vi "LvIRKit_Main.vi"() -> ()   [LabVIEW 2014]
uses:
  <vilib>/Utility/sysdir.llb/System Directory Type.ctl
  <vilib>/Utility/miscctls.llb/LVPointTypeDef.ctl
  <vilib>/Platform/browser.llb/Open URL in Default Browser (string).vi
panel:
  in  "LvIRKit URL":bool
  in  "IRKit URL":bool
  out "title":string="LvIRKit"
  in  "Btn Edit":bool
  in  "Btn Dn":bool
  in  "Btn Up":bool
  in  "Btn Del":bool
  in  "Btn Add":bool
  in  "Btn Enter":bool
  in  "ButtonList":i32(listbox) caption="登録されているリモコンボタン"
  in  "Btn Dev Edit":bool
  in  "Btn Dev Dn":bool
  in  "Btn Dev Up":bool
  in  "Btn Dev Del":bool
  in  "Btn Dev Add":bool
  in  "DeviceList":i32(listbox) caption="IRKit"
  # "IRKit 非公式"
  # "LvIRKitについてはこちら"
  # "IRKitについてはこちら"
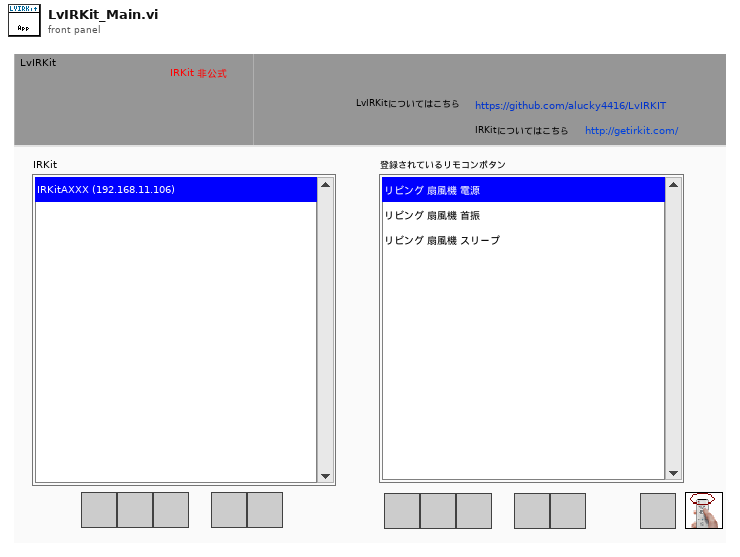
[diagram p1: front panel]
types:
  T1 = enum16{"Init", "Load", "Save", "Get", "Add", "Remove", "Replace", "Up", "Down"}
  T2 = typedef "System Directory Type.ctl" = i32
  T3 = typedef "LvIRKit_rsc_IRData_typedef.ctl" = cluster{"id":i32, "name":string, "irstr":string}
  T4 = typedef "LVPointTypeDef.ctl" = cluster{"Horizontal":i16, "Vertical":i16}
  T5 = cluster{bool, "include Ctrl key?":bool, string}[]
  T6 = enum32{"invalid app kind", "Development System", "Run Time System", "Student Edition", "Embedded LabVIEW", "Evaluation", "Custom"}
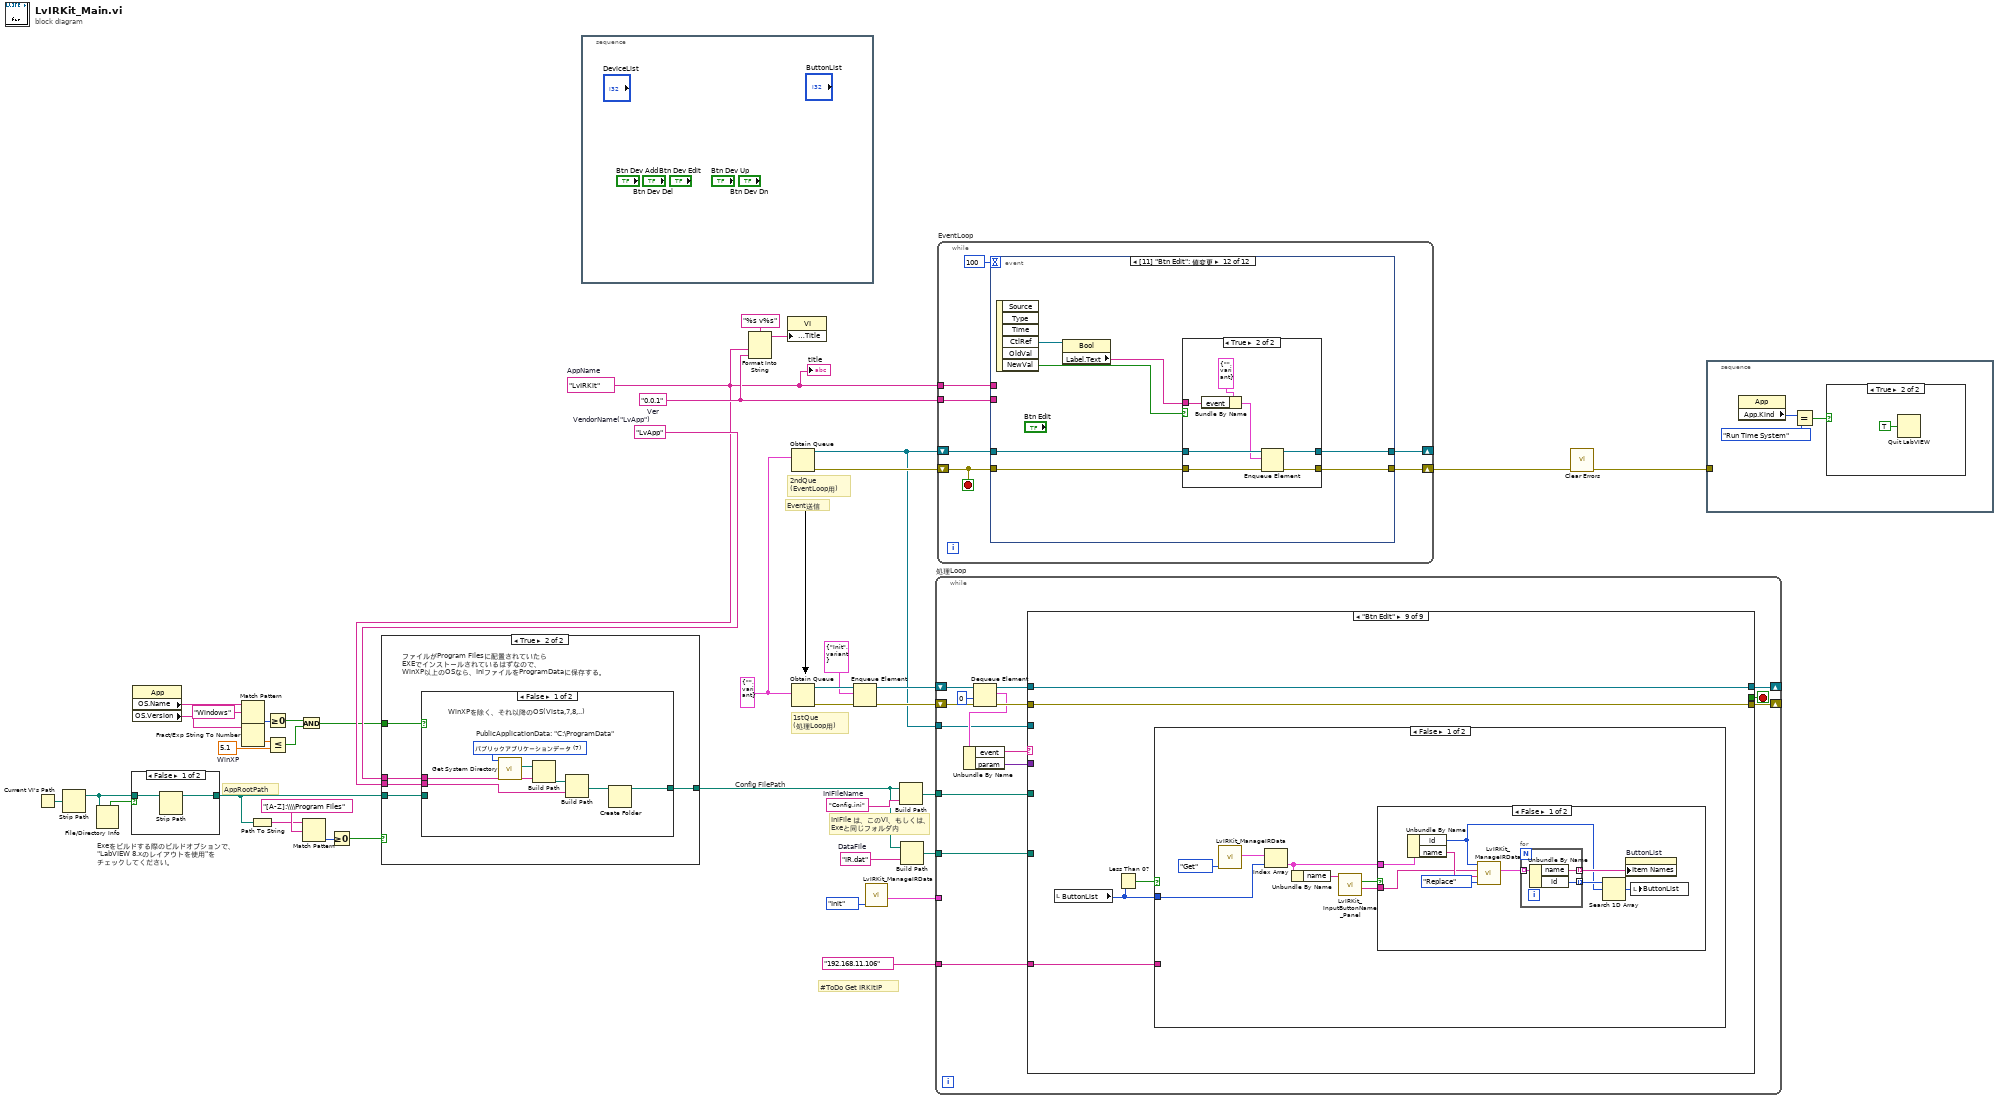
[diagram p0: block diagram]
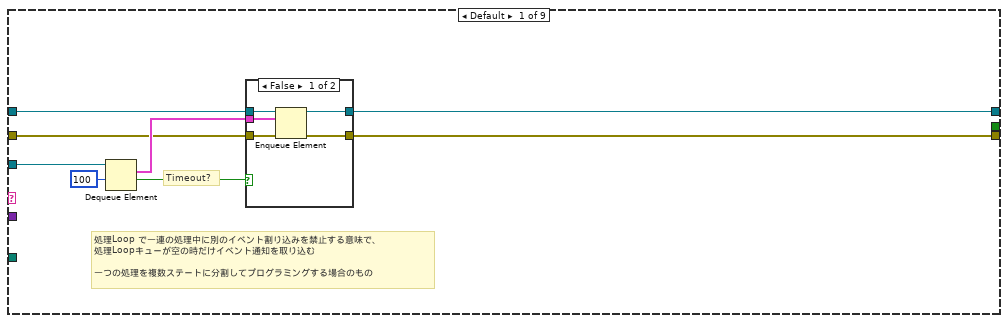
[diagram p6: hidden frame]
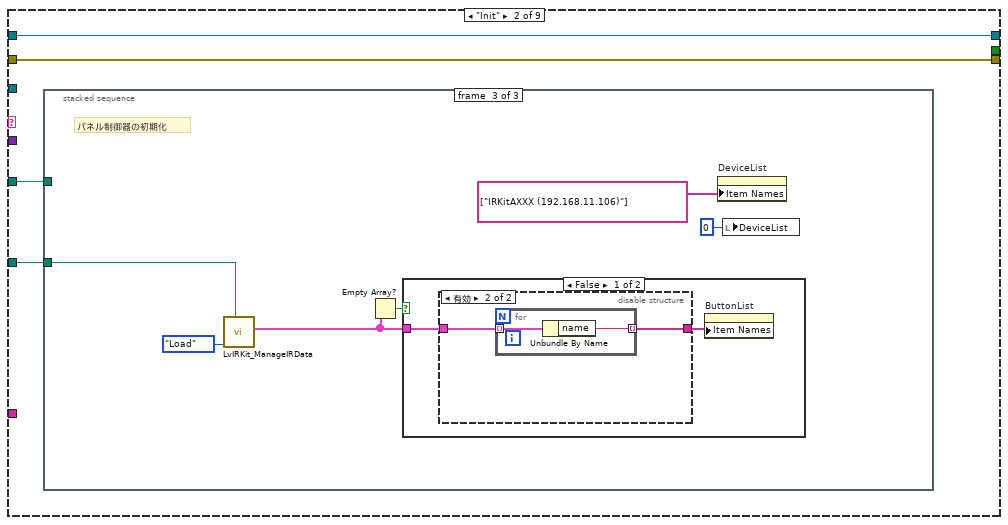
[diagram p8: hidden frame]
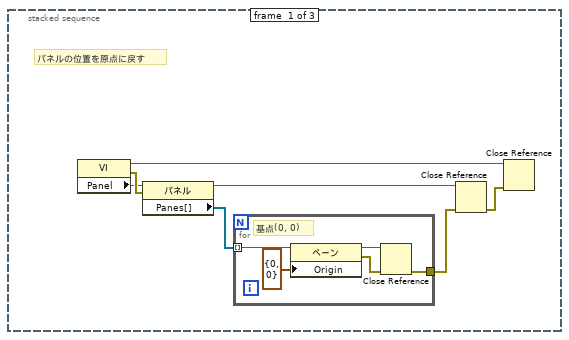
[diagram p9: hidden frame]
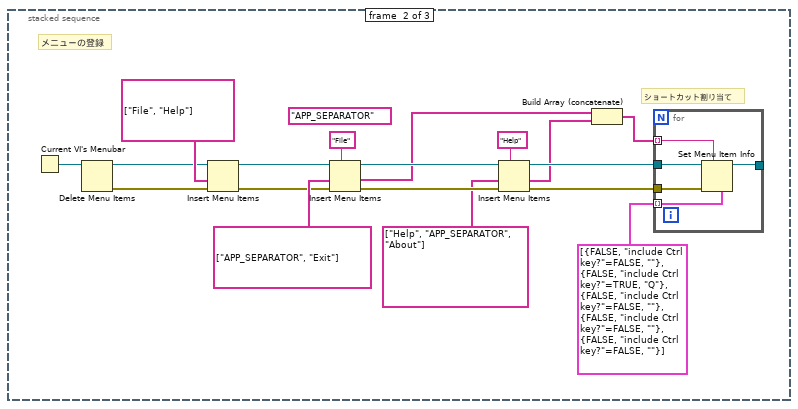
[diagram p10: hidden frame]
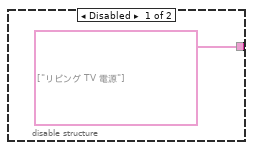
[diagram p11: hidden frame]
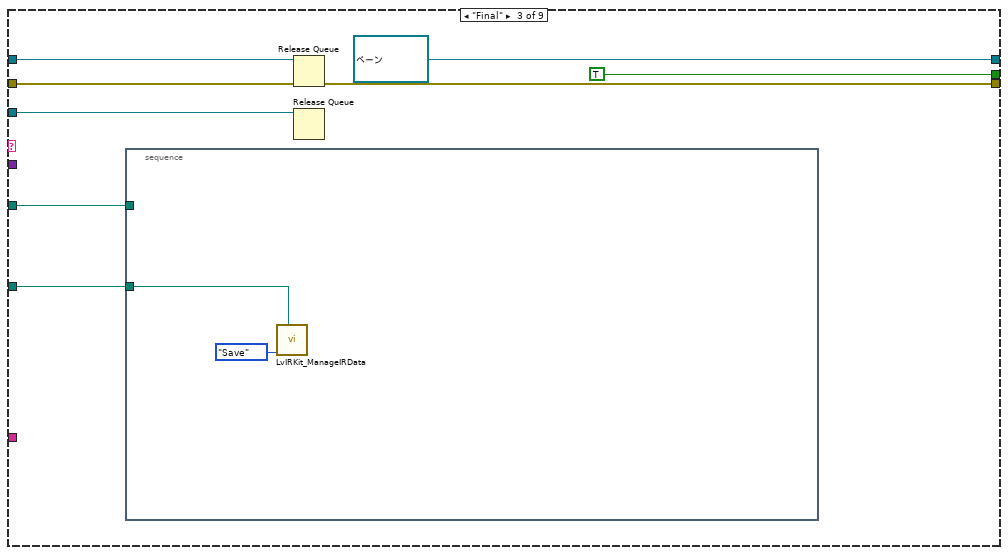
[diagram p13: hidden frame]
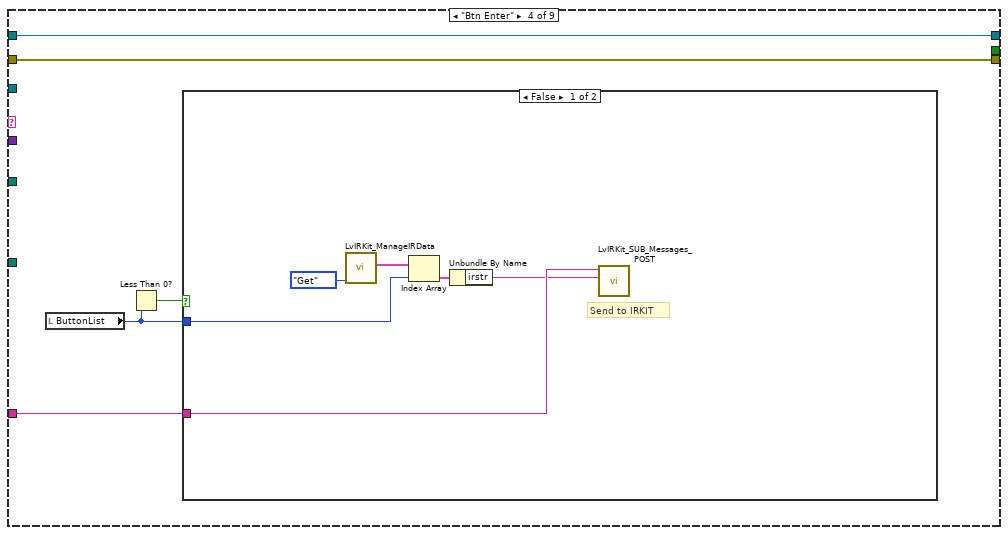
[diagram p14: hidden frame]
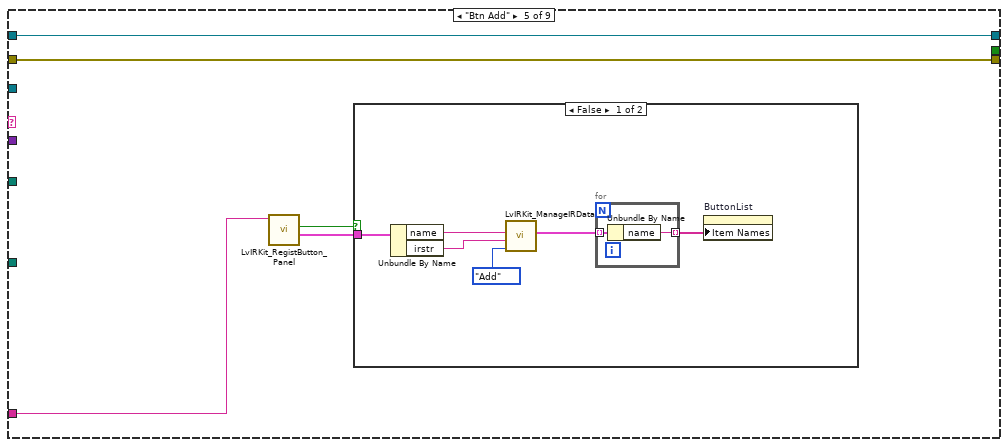
[diagram p16: hidden frame]
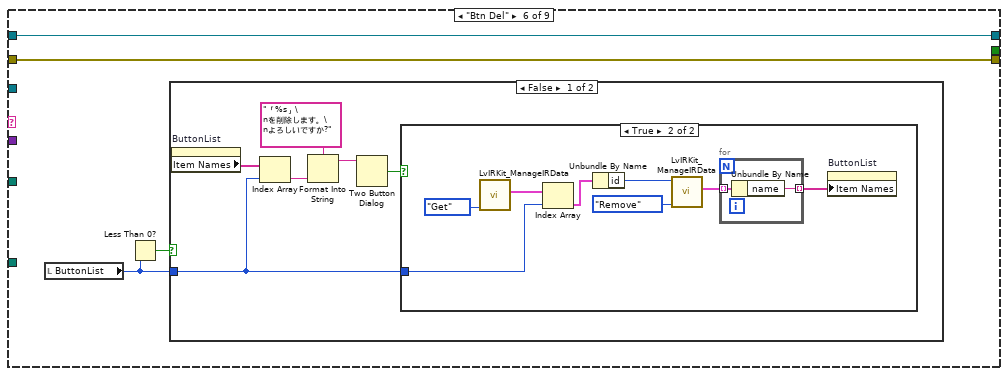
[diagram p18: hidden frame]
diagram:
  w3 = cluster{"event":string, "param":variant} {"event"="", "param"=variant}
  w8 = "IR.dat"  # DataFile
  w19 = "LvApp"  # VendorName("LvApp")
  w23 = 5.1  # WinXP
  w28 = "Config.ini"  # IniFileName
  w31 = "0.0.1"  # Ver
  w18 = "LvIRKit"  # AppName
  # "#ToDo Get IRKitIP"
  # "Exeをビルドする際のビルドオプションで、\n\"LabVIEW 8.xのレイアウトを使用\"を\nチェックしてください。"
  # "Config FilePath"
  # "AppRootPath"
  # "IniFile は、このVI、もしくは、\nExeと同じフォルダ内"
  # "2ndQue\n(EventLoop用)"
  # "1stQue\n(処理Loop用)"
  # "Event送信"
  n1 = Current VI's Path() -> (path=w15:path)
  n2 = Strip Path(path=w15) -> (stripped path=w16:path)  [unwired: 1 out]
  n3 = File/Directory Info(path=w16) -> (directory=w17:bool)  [unwired: 1 in, 6 out]
  n4 = case shown="FALSE" w17 {
    tunnel: w16 -> [w42 w43]
    tunnel: [w41 w43] -> w12
    frame False {
      n5 = Strip Path(path=w42) -> (stripped path=w41:path)  [unwired: 1 out]
    }
    frame True {
    }
  }
  n6 = property class="App"() -> ("OS.Name"=w27:string, "OS.Version"=w25:string)  [unwired: 2 in, 2 out]
  n7 = Match Pattern(string=w27, regular expression="Windows" ("正規表現")) -> (offset past match=w22:i32)  [unwired: 1 in, 3 out]
  n8 = Fract/Exp String To Number(string=w25) -> (number=w24:dbl)  [unwired: 3 in, 1 out]
  n9 = Path To String(path=w12) -> (string=w11:string)
  n10 = Greater Or Equal To 0?(x=w22) -> (x >= 0?=w21:bool)
  n11 = Less Or Equal?(x=w24, y=w23) -> (x <= y?=w20:bool)
  n12 = And(x=w21, y=w20) -> (x .and. y?=w14:bool)
  n13 = Match Pattern(string=w11, regular expression="[A-Z]:\\\\Program Files" ("正規表現")) -> (offset past match=w10:i32)  [unwired: 1 in, 3 out]
  n14 = Greater Or Equal To 0?(x=w10) -> (x >= 0?=w9:bool)
  n15 = case shown="TRUE" w9 {
    tunnel: w18 -> [_ w49]
    tunnel: [w44 w47] -> w7
    tunnel: w19 -> [_ w48]
    tunnel: w14 -> [_ w46]
    tunnel: w12 -> [w44 w45]
    frame False {
      # "ファイルがProgram Filesに配置されていなかったら\n開発システムでソースから実行しているか、\nExeで適当なフォルダから実行されているので、\nIniファイルは、EXE, またはTop VI と同じ場所に保存"
    }
    frame True {
      # "ファイルがProgram Filesに配置されていたら\nEXEでインストールされているはずなので、\nWinXP以上のOSなら、IniファイルをProgramDataに保存する。"
      n16 = case shown="FALSE" w46 {
        tunnel: w49 -> [w53 _]
        tunnel: w48 -> [w51 _]
        tunnel: [w50 w57] -> w47
        tunnel: w45 -> [_ w57]
        frame False {
          w56 = T2 7 items=["ユーザホーム"=0, "ユーザデスクトップ"=1, "ユーザドキュメント"=2, "ユーザアプリケーションデータ"=3, "ユーザ設定"=4, "ユーザ一時"=5, "パブリックドキュメント"=6, "パブリックアプリケーションデータ"=7, "パブリック環境設定"=8, "パブリックキャッシュ"=13, "システムコアライブラリ"=9, "システムインストールされたライブラリ"=10, "アプリケーションファイル"=11, "ブート容量ルート"=12] ("system directory type")
          # "PublicApplicationData: \"C:\\ProgramData\""
          # "WinXPを除く、それ以降のOS(Vista,7,8,..)"
          n17 = call <vilib>:"Get System Directory.vi"("system directory type"=w56) -> ("system directory"=w55:path)  [unwired: 10 in]
          n18 = Build Path(base path=w55, name or relative path=w51) -> (appended path=w54:path)
          n19 = Build Path(base path=w54, name or relative path=w53) -> (appended path=w52:path)
          n20 = Create Folder(path (use dialog)=w52) -> (created path=w50:path)  [unwired: 2 in, 2 out]
        }
        frame True {
        }
      }
    }
  }
  n21 = stacked-sequence {
    frame #0 {
    }
  }
  n22 = Format Into String(format string="%s v%s" ("形式文字列"), w18, w31) -> (resulting string=w29:string)  [unwired: 2 in, 1 out]
  n23 = property class="VI"("Front Panel.Title"=w29) -> ()  [unwired: 2 in, 2 out]
  n24 = Obtain Queue(element data type=w3) -> (queue out=w35:refnum<queue>, error out=w40:errorcluster)  [unwired: 4 in, 1 out]
  n25 = Obtain Queue(element data type=w3) -> (queue out=w39:refnum<queue>, error out=w37:errorcluster)  [unwired: 4 in, 1 out]
  n26 = Enqueue Element(queue=w39, element=cluster{"event":string, "param":variant} {"event"="Init", "param"=variant}, error in (no error)=w37) -> (queue out=w38:refnum<queue>, error out=w36:errorcluster)  [unwired: 1 in, 1 out]
  n27 = call "LvIRKit_ManageIRData.vi"("action"=T1."Init") -> ("irdata out"=w4:T3)  [unwired: 9 in, 1 out]
  n28 = Build Path(base path=w7, name or relative path=w28) -> (appended path=w32:path)
  n29 = Build Path(base path=w7, name or relative path=w8) -> (appended path=w6:path)
  n30 = while "処理Loop" {
    shift-right: [w67] -> _
    shift-left: w38 -> [w72]
    shift-right: [w66] -> _
    shift-left: w36 -> [w69]
    tunnel: w35 -> [w62]
    tunnel: w32 -> [w60]
    tunnel: w6 -> [w59]
    tunnel: w4 -> [_]
    tunnel: "192.168.11.106" ("IRKit IP") -> [w58]
    stop <- w61 stop-if-true
    n31 = Dequeue Element(queue=w72, timeout in ms (-1)=0 ("タイムアウト（ms）（-1）"), error in (no error)=w69) -> (queue out=w71:refnum<queue>, element=w65:cluster{"event":string, "param":variant}, error out=w68:errorcluster)  [unwired: 1 out]
    n32 = Unbundle By Name(w65) -> ("event"=w64:string, "param"=w63:variant)
    n33 = case shown="\"Btn Edit\"" w64 {
      tunnel: w71 -> [w77 w91 w146 w154 w165 w177 w198 w216 w234]
      tunnel: w62 -> [w80 _ w144 _ _ _ _ _ _]
      tunnel: w68 -> [w75 w90 w143 w153 w164 w176 w197 w215 w233]
      tunnel: [w76 w91 refnum<queue> refnum ("queue out") w154 w165 w177 w198 w216 w234] -> w67
      tunnel: [w74 w90 w142 w153 w164 w176 w197 w215 w233] -> w66
      tunnel: w63 -> [_ _ _ _ _ _ _ _ _]
      tunnel: [_ _ TRUE _ _ _ _ _ _] -> w61
      tunnel: w60 -> [_ w89 w141 _ _ _ _ _ _]
      tunnel: w59 -> [_ w88 w140 _ _ _ _ _ _]
      tunnel: w58 -> [_ _ _ w150 w161 _ w194 w212 w230]
      frame Default {
        # "Timeout?"
        # "処理Loop で一連の処理中に別のイベント割り込みを禁止する意味で、\n処理Loopキューが空の時だけイベント通知を取り込む\n\n一つの処理を複数ステートに分割してプログラミングする場合のもの"
        n34 = Dequeue Element(queue=w80, timeout in ms (-1)=100 ("タイムアウト（ms）（-1）")) -> (element=w78:cluster{"event":string, "param":variant}, timed out?=w73:bool)  [unwired: 1 in, 2 out]
        n35 = case shown="FALSE" w73 {
          tunnel: w78 -> [w85 _]
          tunnel: w77 -> [w84 w87]
          tunnel: [w83 w87] -> w76
          tunnel: w75 -> [w82 w86]
          tunnel: [w81 w86] -> w74
          frame False {
            n36 = Enqueue Element(queue=w84, element=w85, error in (no error)=w82) -> (queue out=w83:refnum<queue>, error out=w81:errorcluster)  [unwired: 1 in, 1 out]
          }
          frame True {
          }
        }
      }
      frame "Init" {
        n37 = stacked-sequence {
          tunnel: w89 -> [_ _ _]
          tunnel: w88 -> [_ _ w131]
          frame #0 {
            # "パネルの位置を原点に戻す"
            n38 = property class="VI"() -> (reference out=w95:refnum<vi>, error out=w98:errorcluster, "Panel"=w92:refnum<vi>)  [unwired: 2 in]
            n39 = property on="プロパティノード" class="パネル"(reference=w92, error in=w98) -> (reference out=w94:refnum<vi>, "Panes[]"=w93:refnum<vi>[])  [unwired: 1 out]
            n40 = for {
              tunnel: w93 -> [w103] mode=indexing
              tunnel: [w100] -> w96
              # "基点(0, 0)"
              n41 = property on="プロパティノード" class="ペーン"(reference=w103, "Origin"=T4 {"Horizontal"=0, "Vertical"=0} ("原点")) -> (reference out=w102:refnum<vi>, error out=w101:errorcluster)  [unwired: 1 in]
              n42 = Close Reference(reference=w102, error in (no error)=w101) -> (error out=w100:errorcluster)
            }
            n43 = Close Reference(reference=w94, error in (no error)=w96) -> (error out=w97:errorcluster)
            n44 = Close Reference(reference=w95, error in (no error)=w97) -> ()  [unwired: 1 out]
          }
          frame #1 {
            (unwired) "APP_SEPARATOR"
            # "ショートカット割り当て"
            # "メニューの登録"
            n45 = Current VI's Menubar() -> (w112:refnum<k9>)
            n46 = Delete Menu Items(9:w112) -> (0:w114:errorcluster, 3:w113:refnum<k9>)  [unwired: 3 in]
            n47 = Insert Menu Items(6:w114, 7:string[] ["File", "Help"] ("item tags"), 9:w113) -> (0:w118:errorcluster, 3:w117:refnum<k9>)  [unwired: 3 in, 1 out]
            n48 = Insert Menu Items(5:"File" ("menu tag"), 6:w118, 7:string[] ["APP_SEPARATOR", "Exit"] ("item tags"), 9:w117) -> (0:w121:errorcluster, 1:w107:string[], 3:w120:refnum<k9>)  [unwired: 2 in]
            n49 = Insert Menu Items(5:"Help" ("menu tag"), 6:w121, 7:string[] ["Help", "APP_SEPARATOR", "About"] ("item tags"), 9:w120) -> (0:w108:errorcluster, 1:w106:string[], 3:w109:refnum<k9>)  [unwired: 2 in]
            n50 = Build Array (concatenate)(w107, w106) -> (w104:string[])
            n51 = for {
              tunnel: w109 -> [w126]
              tunnel: w108 -> [w125]
              tunnel: [w124] -> _
              tunnel: T5 [{FALSE, "include Ctrl key?"=FALSE, ""}, {FALSE, "include Ctrl key?"=TRUE, "Q"}, {FALSE, "include Ctrl key?"=FALSE, ""}, {FALSE, "include Ctrl key?"=FALSE, ""}, {FALSE, "include Ctrl key?"=FALSE, ""}] -> [w123] mode=indexing
              tunnel: w104 -> [w122] mode=indexing
              n52 = Set Menu Item Info(4:w123, 7:w122, 8:w125, 11:w126) -> (3:w124:refnum<k9>)  [unwired: 3 in, 1 out]
            }
          }
          frame #2 {
            # "パネル制御器の初期化"
            n53 = call "LvIRKit_ManageIRData.vi"("filepath"=w131, "action"=T1."Load") -> ("IRDATA[]"=w128:T3[])  [unwired: 8 in, 1 out]
            n54 = Empty Array?(array=w128) -> (empty?=w129:bool)
            n55 = case shown="FALSE" w129 {
              tunnel: w128 -> [w133 _]
              frame False {
                n56 = disable-structure shown="有効" {
                  disable-tunnel: [string[] ["リビング TV 電源"] ("項目名") w136] -> w134
                  disable-tunnel: w133 -> [_ w137]
                  frame Disabled {
                  }
                  frame Enabled {
                    n57 = for {
                      tunnel: w137 -> [w139] mode=indexing
                      tunnel: [w138] -> w136 mode=indexing
                      n58 = Unbundle By Name(w139) -> ("name"=w138:string)
                    }
                  }
                }
                n59 = property on="ButtonList" class="LstBox （指定）"("Item Names"=w134) -> ()  [unwired: 2 in, 2 out]
              }
              frame True {
              }
            }
            n60 = property on="DeviceList" class="LstBox （指定）"("Item Names"=string[] ["IRKitAXXX (192.168.11.106)"] ("項目名")) -> ()  [unwired: 2 in, 2 out]
            n61 = local write "DeviceList"(0 ("DeviceList")) -> ()
          }
        }
      }
      frame "Final" {
        n62 = stacked-sequence {
          tunnel: w141 -> [_]
          tunnel: w140 -> [w148]
          frame #0 {
            n63 = call "LvIRKit_ManageIRData.vi"("filepath"=w148, "action"=T1."Save") -> ()  [unwired: 8 in, 2 out]
          }
        }
        n64 = Release Queue(queue=w146, error in (no error)=w143) -> (error out=w142:errorcluster)  [unwired: 1 in, 2 out]
        n65 = Release Queue(queue=w144) -> ()  [unwired: 2 in, 3 out]
      }
      frame "Btn Enter" {
        n66 = local read "ButtonList"() -> (w152:i32)
        n67 = Less Than 0?(x=w152) -> (x < 0?=w151:bool)
        n68 = case shown="FALSE" w151 {
          tunnel: w152 -> [w158 _]
          tunnel: w150 -> [w157 _]
          frame False {
            # "Send to IRKIT"
            n69 = call "LvIRKit_ManageIRData.vi"("action"=T1."Get") -> ("IRDATA[]"=w160:T3[])  [unwired: 9 in, 1 out]
            n70 = Index Array(array=w160, index=w158) -> (element=w156:T3)
            n71 = Unbundle By Name(w156) -> ("irstr"=w155:string)
            n72 = call "LvIRKit_SUB_Messages_POST.vi"("Message"=w155, "IRKit IP address"=w157) -> ()  [unwired: 9 in, 1 out]
          }
          frame True {
          }
        }
      }
      frame "Btn Add" {
        n73 = call "LvIRKit_RegistButton_Panel.vi"("IRKit IP"=w161) -> ("irdata"=w162:T3, "Cancel?"=w163:bool)  [unwired: 9 in]
        n74 = case shown="FALSE" w163 {
          tunnel: w162 -> [w170 _]
          frame False {
            n75 = Unbundle By Name(w170) -> ("name"=w169:string, "irstr"=w168:string)
            n76 = call "LvIRKit_ManageIRData.vi"("action"=T1."Add", "irdata"=w168, "name"=w169) -> ("IRDATA[]"=w166:T3[])  [unwired: 7 in, 1 out]
            n77 = for {
              tunnel: w166 -> [w173] mode=indexing
              tunnel: [w172] -> w167 mode=indexing
              n78 = Unbundle By Name(w173) -> ("name"=w172:string)
            }
            n79 = property on="ButtonList" class="LstBox （指定）"("Item Names"=w167) -> ()  [unwired: 2 in, 2 out]
          }
          frame True {
          }
        }
      }
      frame "Btn Del" {
        n80 = local read "ButtonList"() -> (w175:i32)
        n81 = Less Than 0?(x=w175) -> (x < 0?=w174:bool)
        n82 = case shown="FALSE" w174 {
          tunnel: w175 -> [w178 _]
          frame False {
            n83 = property on="ButtonList" class="LstBox （指定）"() -> ("Item Names"=w183:string[])  [unwired: 2 in, 2 out]
            n84 = Index Array(array=w183, index=w178) -> (element=w182:string)
            n85 = Format Into String(format string="「%s」\nを削除します。\nよろしいですか?" ("メッセージ"), w182) -> (resulting string=w180:string)  [unwired: 2 in, 1 out]
            n86 = Two Button Dialog(message=w180) -> (T button?=w179:bool)  [unwired: 2 in]
            n87 = case shown="TRUE" w179 {
              tunnel: w178 -> [_ w189]
              frame False {
              }
              frame True {
                n88 = call "LvIRKit_ManageIRData.vi"("action"=T1."Get") -> ("IRDATA[]"=w191:T3[])  [unwired: 9 in, 1 out]
                n89 = Index Array(array=w191, index=w189) -> (element=w187:T3)
                n90 = Unbundle By Name(w187) -> ("id"=w186:i32)
                n91 = call "LvIRKit_ManageIRData.vi"("action"=T1."Remove", "id"=w186) -> ("IRDATA[]"=w185:T3[])  [unwired: 8 in, 1 out]
                n92 = for {
                  tunnel: w185 -> [w193] mode=indexing
                  tunnel: [w192] -> w184 mode=indexing
                  n93 = Unbundle By Name(w193) -> ("name"=w192:string)
                }
                n94 = property on="ButtonList" class="LstBox （指定）"("Item Names"=w184) -> ()  [unwired: 2 in, 2 out]
              }
            }
          }
          frame True {
          }
        }
      }
      frame "Btn Up" {
        n95 = local read "ButtonList"() -> (w196:i32)
        n96 = Less Than 0?(x=w196) -> (x < 0?=w195:bool)
        n97 = case shown="FALSE" w195 {
          tunnel: w196 -> [w206 _]
          tunnel: w194 -> [_ _]
          frame False {
            n98 = call "LvIRKit_ManageIRData.vi"("action"=T1."Get") -> ("IRDATA[]"=w208:T3[])  [unwired: 9 in, 1 out]
            n99 = Index Array(array=w208, index=w206) -> (element=w205:T3)
            n100 = Unbundle By Name(w205) -> ("id"=w200:i32)
            n101 = call "LvIRKit_ManageIRData.vi"("action"=T1."Up", "id"=w200) -> ("IRDATA[]"=w202:T3[])  [unwired: 8 in, 1 out]
            n102 = for {
              tunnel: w202 -> [w211] mode=indexing
              tunnel: [w210] -> w203 mode=indexing
              tunnel: [w209] -> w201 mode=indexing
              n103 = Unbundle By Name(w211) -> ("name"=w210:string, "id"=w209:i32)
            }
            n104 = Search 1D Array(1D array=w201, element=w200) -> (index of element=w199:i32)  [unwired: 1 in]
            n105 = property on="ButtonList" class="LstBox （指定）"("Item Names"=w203) -> ()  [unwired: 2 in, 2 out]
            n106 = local write "ButtonList"(w199) -> ()
          }
          frame True {
          }
        }
      }
      frame "Btn Dn" {
        n107 = local read "ButtonList"() -> (w214:i32)
        n108 = Less Than 0?(x=w214) -> (x < 0?=w213:bool)
        n109 = case shown="FALSE" w213 {
          tunnel: w214 -> [w224 _]
          tunnel: w212 -> [_ _]
          frame False {
            n110 = call "LvIRKit_ManageIRData.vi"("action"=T1."Get") -> ("IRDATA[]"=w226:T3[])  [unwired: 9 in, 1 out]
            n111 = Index Array(array=w226, index=w224) -> (element=w223:T3)
            n112 = Unbundle By Name(w223) -> ("id"=w218:i32)
            n113 = call "LvIRKit_ManageIRData.vi"("action"=T1."Down", "id"=w218) -> ("IRDATA[]"=w220:T3[])  [unwired: 8 in, 1 out]
            n114 = for {
              tunnel: w220 -> [w229] mode=indexing
              tunnel: [w228] -> w221 mode=indexing
              tunnel: [w227] -> w219 mode=indexing
              n115 = Unbundle By Name(w229) -> ("name"=w228:string, "id"=w227:i32)
            }
            n116 = Search 1D Array(1D array=w219, element=w218) -> (index of element=w217:i32)  [unwired: 1 in]
            n117 = property on="ButtonList" class="LstBox （指定）"("Item Names"=w221) -> ()  [unwired: 2 in, 2 out]
            n118 = local write "ButtonList"(w217) -> ()
          }
          frame True {
          }
        }
      }
      frame "Btn Edit" {
        n119 = local read "ButtonList"() -> (w232:i32)
        n120 = Less Than 0?(x=w232) -> (x < 0?=w231:bool)
        n121 = case shown="FALSE" w231 {
          tunnel: w232 -> [w241 _]
          tunnel: w230 -> [_ _]
          frame False {
            n122 = call "LvIRKit_ManageIRData.vi"("action"=T1."Get") -> ("IRDATA[]"=w240:T3[])  [unwired: 9 in, 1 out]
            n123 = Index Array(array=w240, index=w241) -> (element=w236:T3)
            n124 = Unbundle By Name(w236) -> ("name"=w238:string)
            n125 = call "LvIRKit_InputButtonName_Panel.vi"("button name"=w238) -> ("buttunName"=w237:string, "Cancel?"=w235:bool)  [unwired: 9 in]
            n126 = case shown="FALSE" w235 {
              tunnel: w237 -> [w243 _]
              tunnel: w236 -> [w242 _]
              frame False {
                n127 = Unbundle By Name(w242) -> ("id"=w245:i32, "name"=w244:string)
                n128 = call "LvIRKit_ManageIRData.vi"("action"=T1."Replace", "irdata"=w244, "name"=w243, "id"=w245) -> ("IRDATA[]"=w249:T3[])  [unwired: 6 in, 1 out]
                n129 = for {
                  tunnel: w249 -> [w253] mode=indexing
                  tunnel: [w252] -> w250 mode=indexing
                  tunnel: [w251] -> w248 mode=indexing
                  n130 = Unbundle By Name(w253) -> ("name"=w252:string, "id"=w251:i32)
                }
                n131 = Search 1D Array(1D array=w248, element=w245) -> (index of element=w247:i32)  [unwired: 1 in]
                n132 = property on="ButtonList" class="LstBox （指定）"("Item Names"=w250) -> ()  [unwired: 2 in, 2 out]
                n133 = local write "ButtonList"(w247) -> ()
              }
              frame True {
              }
            }
          }
          frame True {
          }
        }
      }
    }
  }
  n134 = while "EventLoop" {
    shift-right: [w258] -> _
    shift-left: w35 -> [w259]
    shift-right: [w257] -> w34
    shift-left: w40 -> [w256]
    tunnel: w18 -> [w255]
    tunnel: w31 -> [w254]
    stop <- w256 stop-if-true
    n135 = event shown="[11] \"Btn Edit\": 値変更" {
      selector: _ -> [_ _ _ _ _ _ _ _ _ _ _ _]
      dyn-events: _ -> [_ _ _ _ _ _ _ _ _ _ _ _]
      timeout: 100 -> [_ _ _ _ _ _ _ _ _ _ _ _]
      tunnel: w259 -> [w264 w270 w276 w280 w284 w292 w314 w330 w346 w362 w378 w394]
      tunnel: [w261 w269 w275 w280 w284 w291 w313 w329 w345 w361 w377 w393] -> w258
      tunnel: w256 -> [w263 w268 w274 w279 w283 w290 w312 w328 w344 w360 w376 w392]
      tunnel: [w262 w267 w273 w279 w283 w289 w311 w327 w343 w359 w375 w391] -> w257
      tunnel: w255 -> [_ _ _ _ _ w287 _ _ _ _ _ _]
      tunnel: w254 -> [_ _ _ _ _ w286 _ _ _ _ _ _]
      event Timeout {
        # "EventLoopの終了用"
        # "Que解放をチェック\n(終了?)"
        n136 = event-data() -> ()  [unwired: 1 in, 2 out]
        n137 = Get Queue Status(queue=w264, error in (no error)=w263) -> (queue out=w261:refnum<queue>, error out=w262:errorcluster)  [unwired: 1 in, 6 out]
      }
      event Application Instance Close? {
        n138 = event-data() -> ()  [unwired: 1 in, 4 out]
        n139 = Enqueue Element(queue=w270, element=cluster{"event":string, "param":variant} {"event"="Final", "param"=variant}, error in (no error)=w268) -> (queue out=w269:refnum<queue>, error out=w267:errorcluster)  [unwired: 1 in, 1 out]
        n140 = event-data("SilentShutdown"=TRUE, "Discard?"=FALSE ("破棄?")) -> ()  [unwired: 1 in, 1 out]
      }
      event Panel Close? {
        n141 = event-data() -> ()  [unwired: 1 in, 3 out]
        n142 = Enqueue Element(queue=w276, element=cluster{"event":string, "param":variant} {"event"="Final", "param"=variant}, error in (no error)=w274) -> (queue out=w275:refnum<queue>, error out=w273:errorcluster)  [unwired: 1 in, 1 out]
        n143 = event-data("Discard?"=TRUE) -> ()  [unwired: 1 in, 1 out]
      }
      event "IRKit URL": Value Change {
        n144 = event-data() -> ("CtlRef"=w281:refnum<vi>)  [unwired: 1 in, 5 out]
        n145 = property class="Bool"(reference=w281) -> ("BoolText.Text"=w278:string)  [unwired: 1 in, 2 out]
        n146 = call-poly <vilib>:"Open URL in Default Browser.vi"("URL"=w278) -> ()  [unwired: 5 in, 2 out]
      }
      event "LvIRKit URL": Value Change {
        n147 = event-data() -> ("CtlRef"=w285:refnum<vi>)  [unwired: 1 in, 5 out]
        n148 = property class="Bool"(reference=w285) -> ("BoolText.Text"=w282:string)  [unwired: 1 in, 2 out]
        n149 = call-poly <vilib>:"Open URL in Default Browser.vi"("URL"=w282) -> ()  [unwired: 5 in, 2 out]
      }
      event Menu Selection (User) {
        n150 = event-data() -> ("ItemPath"=w288:string)  [unwired: 1 in, 5 out]
        n151 = case shown="デフォルト" w288 {
          tunnel: w292 -> [w294 w299 w305 w307]
          tunnel: [w294 w298 w305 w307] -> w291
          tunnel: w290 -> [w293 w297 w304 w306]
          tunnel: [w293 w296 w304 w306] -> w289
          tunnel: w287 -> [_ _ w303 _]
          tunnel: w286 -> [_ _ w302 _]
          frame Default {
          }
          frame "File:Exit" {
            n152 = Enqueue Element(queue=w299, element=cluster{string, "バリアント":variant} {"Final", "バリアント"=variant}, error in (no error)=w297) -> (queue out=w298:refnum<queue>, error out=w296:errorcluster)  [unwired: 1 in, 1 out]
          }
          frame "Help:About" {
            n153 = Format Into String(format string="%s\n\nVersion : %s" ("メッセージ"), w303, w302) -> (resulting string=w300:string)  [unwired: 2 in, 1 out]
            n154 = One Button Dialog(message=w300) -> ()  [unwired: 1 in, 1 out]
          }
          frame "Help:Help" {
          }
        }
      }
      event "Btn Enter": Value Change {
        n155 = event-data() -> ("CtlRef"=w310:refnum<vi>, "NewVal"=w308:bool)  [unwired: 1 in, 4 out]
        n156 = property class="Bool"(reference=w310) -> ("Label.Text"=w309:string)  [unwired: 1 in, 2 out]
        n157 = case shown="TRUE" w308 {
          tunnel: w314 -> [w316 w323]
          tunnel: [w316 w322] -> w313
          tunnel: w312 -> [w315 w321]
          tunnel: [w315 w320] -> w311
          tunnel: w309 -> [_ w318]
          frame False {
          }
          frame True {
            n158 = Bundle By Name(cluster=cluster{"event":string, "param":variant} {"event"="", "param"=variant}, "event"=w318) -> (w317:cluster{"event":string, "param":variant})
            n159 = Enqueue Element(queue=w323, element=w317, error in (no error)=w321) -> (queue out=w322:refnum<queue>, error out=w320:errorcluster)  [unwired: 1 in, 1 out]
          }
        }
      }
      event "Btn Add": Value Change {
        n160 = event-data() -> ("CtlRef"=w326:refnum<vi>, "NewVal"=w324:bool)  [unwired: 1 in, 4 out]
        n161 = property class="Bool"(reference=w326) -> ("Label.Text"=w325:string)  [unwired: 1 in, 2 out]
        n162 = case shown="TRUE" w324 {
          tunnel: w330 -> [w332 w339]
          tunnel: [w332 w338] -> w329
          tunnel: w328 -> [w331 w337]
          tunnel: [w331 w336] -> w327
          tunnel: w325 -> [_ w334]
          frame False {
          }
          frame True {
            n163 = Bundle By Name(cluster=cluster{"event":string, "param":variant} {"event"="", "param"=variant}, "event"=w334) -> (w333:cluster{"event":string, "param":variant})
            n164 = Enqueue Element(queue=w339, element=w333, error in (no error)=w337) -> (queue out=w338:refnum<queue>, error out=w336:errorcluster)  [unwired: 1 in, 1 out]
          }
        }
      }
      event "Btn Up": Value Change {
        n165 = event-data() -> ("CtlRef"=w342:refnum<vi>, "NewVal"=w340:bool)  [unwired: 1 in, 4 out]
        n166 = property class="Bool"(reference=w342) -> ("Label.Text"=w341:string)  [unwired: 1 in, 2 out]
        n167 = case shown="TRUE" w340 {
          tunnel: w346 -> [w348 w355]
          tunnel: [w348 w354] -> w345
          tunnel: w344 -> [w347 w353]
          tunnel: [w347 w352] -> w343
          tunnel: w341 -> [_ w350]
          frame False {
          }
          frame True {
            n168 = Bundle By Name(cluster=cluster{"event":string, "param":variant} {"event"="", "param"=variant}, "event"=w350) -> (w349:cluster{"event":string, "param":variant})
            n169 = Enqueue Element(queue=w355, element=w349, error in (no error)=w353) -> (queue out=w354:refnum<queue>, error out=w352:errorcluster)  [unwired: 1 in, 1 out]
          }
        }
      }
      event "Btn Dn": Value Change {
        n170 = event-data() -> ("CtlRef"=w358:refnum<vi>, "NewVal"=w356:bool)  [unwired: 1 in, 4 out]
        n171 = property class="Bool"(reference=w358) -> ("Label.Text"=w357:string)  [unwired: 1 in, 2 out]
        n172 = case shown="TRUE" w356 {
          tunnel: w362 -> [w364 w371]
          tunnel: [w364 w370] -> w361
          tunnel: w360 -> [w363 w369]
          tunnel: [w363 w368] -> w359
          tunnel: w357 -> [_ w366]
          frame False {
          }
          frame True {
            n173 = Bundle By Name(cluster=cluster{"event":string, "param":variant} {"event"="", "param"=variant}, "event"=w366) -> (w365:cluster{"event":string, "param":variant})
            n174 = Enqueue Element(queue=w371, element=w365, error in (no error)=w369) -> (queue out=w370:refnum<queue>, error out=w368:errorcluster)  [unwired: 1 in, 1 out]
          }
        }
      }
      event "Btn Del": Value Change {
        n175 = event-data() -> ("CtlRef"=w374:refnum<vi>, "NewVal"=w372:bool)  [unwired: 1 in, 4 out]
        n176 = property class="Bool"(reference=w374) -> ("Label.Text"=w373:string)  [unwired: 1 in, 2 out]
        n177 = case shown="TRUE" w372 {
          tunnel: w378 -> [w380 w387]
          tunnel: [w380 w386] -> w377
          tunnel: w376 -> [w379 w385]
          tunnel: [w379 w384] -> w375
          tunnel: w373 -> [_ w382]
          frame False {
          }
          frame True {
            n178 = Bundle By Name(cluster=cluster{"event":string, "param":variant} {"event"="", "param"=variant}, "event"=w382) -> (w381:cluster{"event":string, "param":variant})
            n179 = Enqueue Element(queue=w387, element=w381, error in (no error)=w385) -> (queue out=w386:refnum<queue>, error out=w384:errorcluster)  [unwired: 1 in, 1 out]
          }
        }
      }
      event "Btn Edit": Value Change {
        n180 = event-data() -> ("CtlRef"=w390:refnum<vi>, "NewVal"=w388:bool)  [unwired: 1 in, 4 out]
        n181 = property class="Bool"(reference=w390) -> ("Label.Text"=w389:string)  [unwired: 1 in, 2 out]
        n182 = case shown="TRUE" w388 {
          tunnel: w394 -> [w396 w403]
          tunnel: [w396 w402] -> w393
          tunnel: w392 -> [w395 w401]
          tunnel: [w395 w400] -> w391
          tunnel: w389 -> [_ w398]
          frame False {
          }
          frame True {
            n183 = Bundle By Name(cluster=cluster{"event":string, "param":variant} {"event"="", "param"=variant}, "event"=w398) -> (w397:cluster{"event":string, "param":variant})
            n184 = Enqueue Element(queue=w403, element=w397, error in (no error)=w401) -> (queue out=w402:refnum<queue>, error out=w400:errorcluster)  [unwired: 1 in, 1 out]
          }
        }
      }
    }
  }
  n185 = call <vilib>:"Clear Errors.vi"("error in (no error)"=w34) -> ("error out"=w33:errorcluster)  [unwired: 5 in, 1 out]
  n186 = stacked-sequence {
    tunnel: w33 -> [_]
    frame #0 {
      n187 = property class="App"() -> ("App.Kind"=w406:T6)  [unwired: 2 in, 2 out]
      n188 = Equal?(x=w406, y=T6."Run Time System" ("アプリケーション:種類")) -> (x = y?=w404:bool)
      n189 = case shown="TRUE" w404 {
        frame False {
        }
        frame True {
          n190 = Quit LabVIEW(quit? (T)=TRUE ("終了?（T）")) -> ()
        }
      }
    }
  }
  "title" <- w18
